vi "Open_Image.vi"(11 "NewVal":path) -> (3 "image data":T1)   [LabVIEW 2020]
uses:
  <vilib>/picture/picture.llb/imagedata.ctl
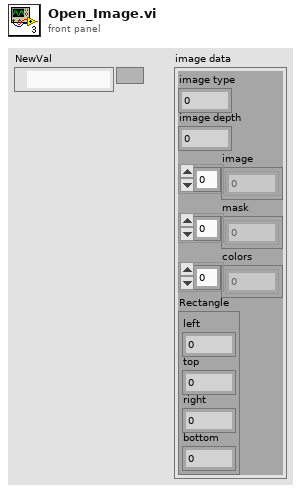
[diagram p1: front panel]
types:
  T1 = typedef "imagedata.ctl" = cluster{"image type":i32, "image depth":i32, "image":u8[], "mask":u8[], "colors":u32[], "Rectangle":cluster{"left":i16, "top":i16, "right":i16, "bottom":i16}}
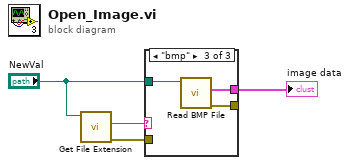
[diagram p0: block diagram]
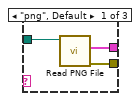
[diagram p2: hidden frame]
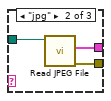
[diagram p3: hidden frame]
diagram:
  n1 = call <vilib>:"Get File Extension.vi"("file"="NewVal") -> ("error out"=w4:errorcluster, "lowercase file extension"=w2:string)  [unwired: 6 in, 3 out]
  n2 = case shown="\"bmp\"" w2 {
    tunnel: [w7 w10 w13] -> w1
    tunnel: "NewVal" -> [w6 w9 w12]
    tunnel: w4 -> [_ _ _]
    tunnel: [w5 w8 w11] -> _
    frame "png", Default {
      n3 = call <vilib>:"Read PNG File.vi"("path to PNG file"=w6) -> ("error out"=w5:errorcluster, "image data"=w7:T1)  [unwired: 8 in, 1 out]
    }
    frame "jpg" {
      n4 = call <vilib>:"Read JPEG File.vi"("path to JPEG file"=w9) -> ("error out"=w8:errorcluster, "image data"=w10:T1)  [unwired: 8 in, 1 out]
    }
    frame "bmp" {
      n5 = call <vilib>:"Read BMP File.vi"("path to BMP file"=w12) -> ("error out"=w11:errorcluster, "image data"=w13:T1)  [unwired: 8 in, 1 out]
    }
  }
  "image data" <- w1
